vi "Set Series CFG.vi"(8 "error in (no error)":errorcluster, 10 "Study CFG":string, 11 "HAL GOOP4:Series Base in":refnum<class "Series Base.lvclass">) -> (0 "error out":errorcluster, 3 "HAL GOOP4:Series Base out":refnum<class "Series Base.lvclass">)   [LabVIEW 2023, in "HAL GOOP4.lvlib" / "Series Base.lvclass"]
uses:
  Series Base.lvclass
  Series Base.lvclass/Series Base.ctl
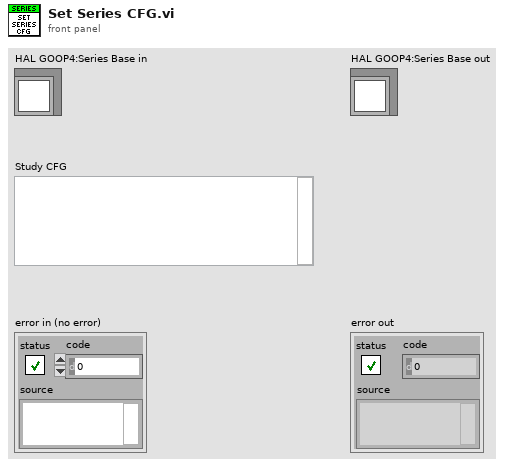
[diagram p1: front panel]
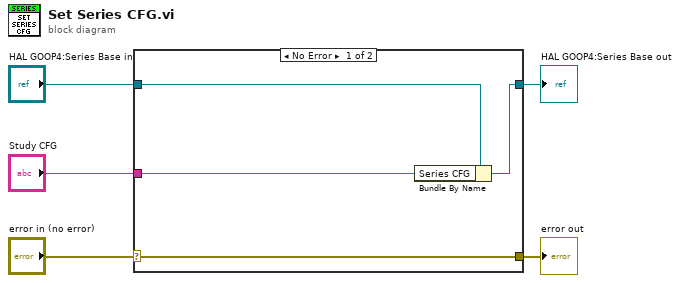
[diagram p0: block diagram]
diagram:
  n1 = case shown="No Error" "error in (no error)" {
    selector: "error in (no error)" -> [w9 w10]
    tunnel: [w9 w10] -> w4
    tunnel: [w7 w11] -> w2
    tunnel: "HAL GOOP4:Series Base in" -> [w8 w11]
    tunnel: "Study CFG" -> [w6 _]
    frame No Error {
      n2 = Bundle By Name(cluster=w8, "Series CFG"=w6) -> (w7:refnum<class "Series Base.lvclass">)
    }
    frame Error {
    }
  }
  "error out" <- w4
  "HAL GOOP4:Series Base out" <- w2
